vi "Fetch Acquired Data (U16).vi"(7 "Timeout (s)":i32=5, 8 "error out":errorcluster, 10 "Samples":i32=-1, 11 "FPGA Ref In":refnum<k20>) -> (0 "error out":errorcluster, 2 "Data":i16[](array[numeric]), 3 "FPGA RefOut":refnum<k20>, 4 "Elements Remaining":u32)   [LabVIEW 2012]
uses:
  <vilib>/Utility/error.llb/Error Cluster From Error Code.vi
  <vilib>/rvi/errors/niLvFpgaAdjustHostInterfaceError.vi
  <vilib>/rvi/interface/nirviMethod/nirviMethod.xnode
  <vilib>/rvi/errors/niLvFpgaMergeErrorWithErrorCode.vi
  <vilib>/FPGAPlugInAG/Dynamic/niLvFpga_ReadFifo_Dynamic.vi
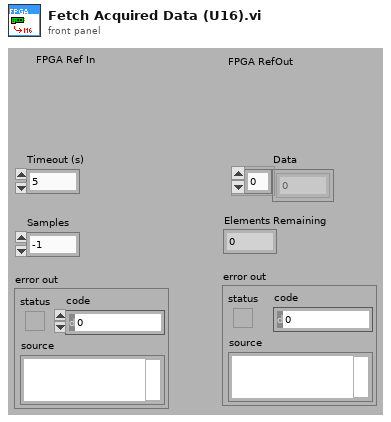
[diagram p1: front panel]
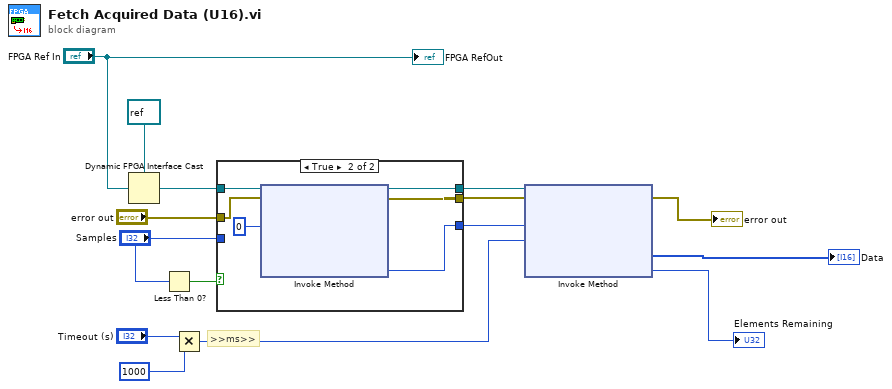
[diagram p0: block diagram]
diagram:
  # ">>ms>>"
  n1 = Dynamic FPGA Interface Cast(Session In=refnum<k20> refnum ("Type"), Type="FPGA Ref In") -> (Session Out=w2:refnum<k20>)
  n2 = Less Than 0?(x="Samples") -> (x < 0?=w12:bool)
  n3 = Multiply(x="Timeout (s)", y=1000) -> (x*y=w6:i32)
  n4 = case shown="True" w12 {
    tunnel: w2 -> [w18 w24]
    tunnel: "error out" -> [w17 w23]
    tunnel: [w18 w22] -> w10
    tunnel: [w17 w21] -> w9
    tunnel: [w16 w19] -> w7
    tunnel: "Samples" -> [w16 _]
    frame False {
    }
    frame True {
      n5 = xnode "Invoke Method"("FPGA VI Reference In"=w24, "error in"=w23, "Number of Elements"=u32 0) -> ("FPGA VI Reference Out"=w22:refnum<k20>, "error out"=w21:errorcluster, "Elements Remaining"=w19:u32)  [unwired: 1 in, 1 out]
    }
  }
  n6 = xnode "Invoke Method"("FPGA VI Reference In"=w10, "error in"=w9, "Number of Elements"=w7, "Timeout (ms)"=w6) -> ("error out"=→"error out":errorcluster, "Data"=→"Data":i16[], "Elements Remaining"=→"Elements Remaining":u32)  [unwired: 1 out]
  "FPGA RefOut" <- "FPGA Ref In"
